vi "Gather Control References.vi"(8 "error in (no error)":errorcluster, 11 "Rename in":refnum<class "Rename.lvclass">) -> (0 "error out":errorcluster, 3 "Rename out":refnum<class "Rename.lvclass">)   [LabVIEW 2015, in "Generic Module Library.lvlib" / "Template G_Module.lvlib" / "Rename.lvclass"]
uses:
  Rename.lvclass
  Private API/Module Control Manager/Control_Mgr_Class/Controls_Mgr.lvclass
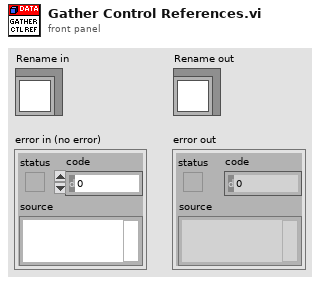
[diagram p1: front panel]
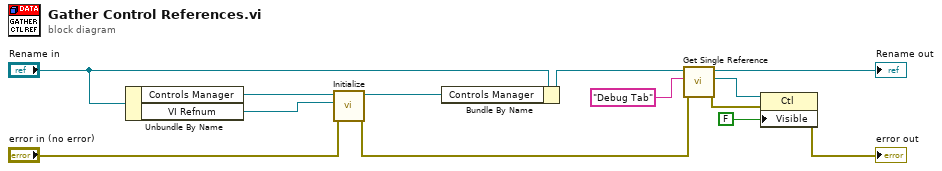
[diagram p0: block diagram]
diagram:
  n1 = Unbundle By Name("Rename in") -> ("Controls Manager"=w11:refnum<class "Controls_Mgr.lvclass">, "VI Refnum"=w10:refnum<vi>)
  n2 = call-dynamic "Initialize.vi"("error in"="error in (no error)", "VI Refnum"=w10, "ManageControls in"=w11) -> ("error out"=w1:errorcluster, "ManageControls out"=w9:refnum<class "Controls_Mgr.lvclass">)  [unwired: 7 in]
  n3 = Bundle By Name(cluster="Rename in", "Controls Manager"=w9) -> (w5:refnum<class "Rename.lvclass">)
  n4 = call "Get Single Reference.vi"("error in (no error)"=w1, "Control Name"="Debug Tab", "Rename in"=w5) -> ("error out"=w6:errorcluster, "Control Reference"=w7:refnum<vi>, "Rename out"=→"Rename out":refnum<class "Rename.lvclass">)  [unwired: 6 in]
  n5 = property class="Ctl"(reference=w7, error in=w6, "Visible"=FALSE) -> (error out=→"error out":errorcluster)  [unwired: 1 out]
